vi "Save to CSV.vi"(8 "error in (no error)":errorcluster, 11 "Scan Data Process":T1) -> (0 "error out":errorcluster, 3 "Scan Data Process out":T1)   [LabVIEW 2015, in "Exposure Process.lvlib"]
uses:
  Exposure Process.lvlib
  Control_Scan Data Process.ctl
  <vilib>/addons/PointValueMap/controls/PointMap.ctl
  Control_EXP Information.ctl
  Control_File Save Setup.ctl
  Control_Enable and Path.ctl
  Control_ICM Export Setting.ctl
  FileHandler/controls/Record.ctl
  <vilib>/Utility/file.llb/Write Delimited Spreadsheet (string).vi
  FileHandler/FileHandler.lvlib
  <vilib>/addons/PointValueMap/PointValueMap.lvlib
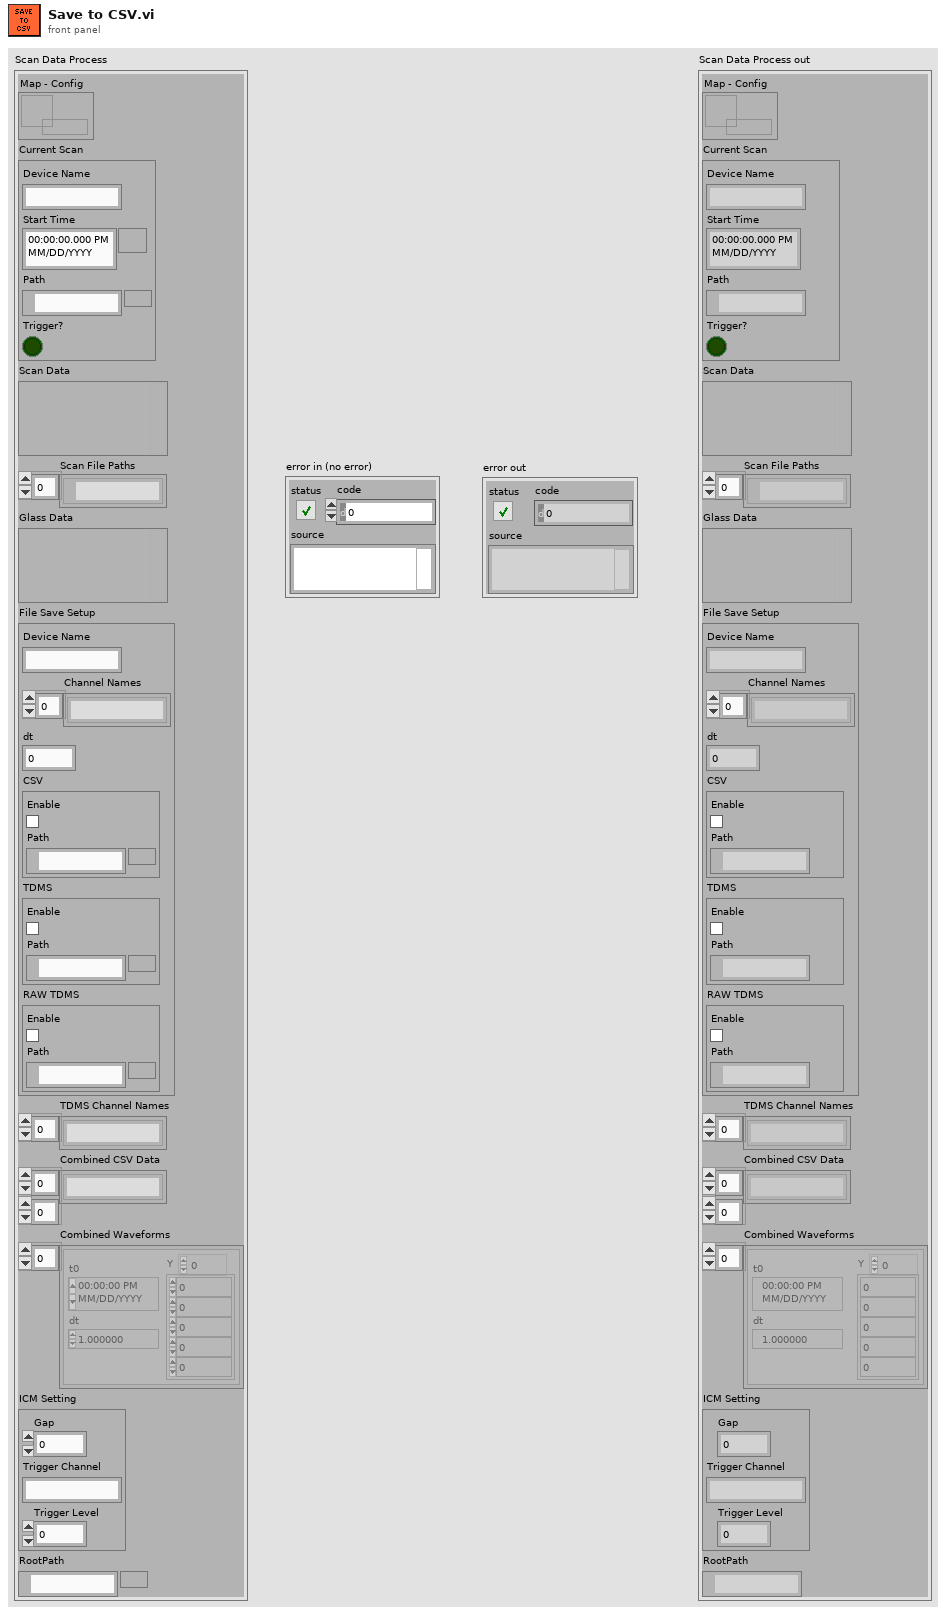
[diagram p1: front panel]
types:
  T1 = typedef "Exposure Process.lvlib/Control_Scan Data Process.ctl" = cluster{"Map - Config":T2, "Current Scan":T3, "Scan Data":variant, "Scan File Paths":path[], "Glass Data":variant, "File Save Setup":T4, "TDMS Channel Names":string[], "Combined CSV Data":string[][], "Combined Waveforms":waveform(dbl)[], "ICM Setting":T6, "RootPath":path}
  T2 = typedef "PointValueMap.lvlib/PointMap.ctl" = refnum<data-value>
  T3 = typedef "Exposure Process.lvlib/Control_EXP Information.ctl" = cluster{"Device Name":string, "Start Time":timestamp, "Path":path, "Trigger?":bool}
  T4 = typedef "Exposure Process.lvlib/Control_File Save Setup.ctl" = cluster{"Device Name":string, "Channel Names":string[], "dt":dbl, "CSV":T5, "TDMS":T5, "RAW TDMS":T5}
  T5 = typedef "Exposure Process.lvlib/Control_Enable and Path.ctl" = cluster{"Enable":bool, "Path":path}
  T6 = typedef "Exposure Process.lvlib/Control_ICM Export Setting.ctl" = cluster{"Gap":dbl, "Trigger Channel":string, "Trigger Level":dbl}
  T7 = typedef "FileHandler.lvlib/Record.ctl" = cluster{"Time":timestamp, "Path":path}
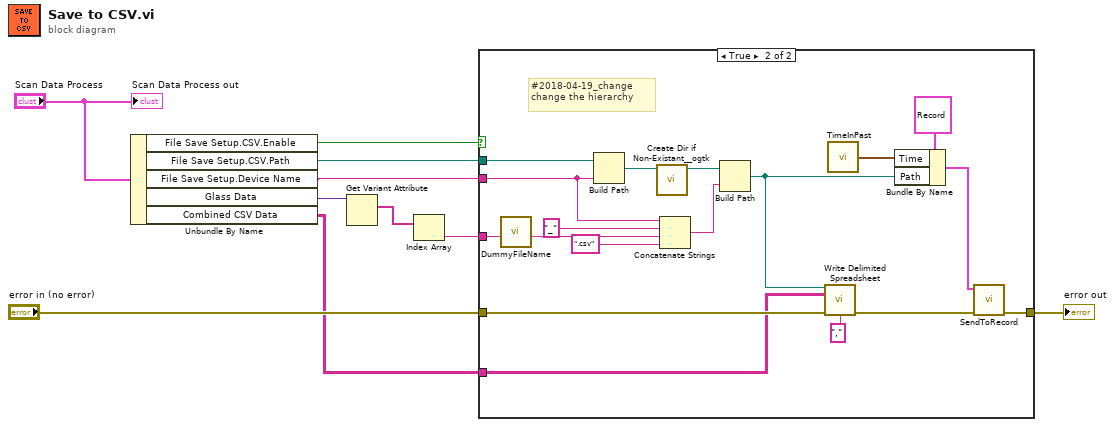
[diagram p0: block diagram]
diagram:
  n1 = Unbundle By Name("Scan Data Process") -> ("File Save Setup.CSV.Enable"=w9:bool, "File Save Setup.CSV.Path"=w8:path, "File Save Setup.Device Name"=w7:string, "Glass Data"=w4:variant, "Combined CSV Data"=w5:string[][])
  n2 = Get Variant Attribute(Variant=w4) -> (names=w3:string[])  [unwired: 3 in, 3 out]
  n3 = Index Array(array=w3) -> (element=w2:string)  [unwired: 1 in]
  n4 = case shown="True" w9 {
    tunnel: w2 -> [_ w14]
    tunnel: "error in (no error)" -> [w11 w25]
    tunnel: [w11 w18] -> w10
    tunnel: w5 -> [_ w23]
    tunnel: w8 -> [_ w22]
    tunnel: w7 -> [_ w20]
    frame False {
    }
    frame True {
      # "#2018-04-19_change\nchange the hierarchy"
      n5 = call "DummyFileName.vi"("Time String in"=w14) -> ("Time String out"=w13:string)  [unwired: 9 in, 1 out]
      n6 = Build Path(base path=w22, name or relative path=w20) -> (appended path=w21:path)
      n7 = call <userlib>:"Create Dir if Non-Existant__ogtk.vi"("Directory Path"=w21) -> ("dup Directory Path"=w26:path)  [unwired: 8 in, 2 out]
      n8 = Concatenate Strings(w20, "_" ("string"), w13, ".csv" ("string")) -> (w27:string)
      n9 = Build Path(base path=w26, name or relative path=w27) -> (appended path=w16:path)
      n10 = call-poly <vilib>:"Write Delimited Spreadsheet.vi"("file path (dialog if empty)"=w16, "2D data"=w23, "error in (no error)"=w25, "delimiter (\\t)"="," ("delimiter (\\t)")) -> ("error out"=w19:errorcluster)  [unwired: 10 in, 1 out]
      n11 = call "TimeInPast.vi"() -> ("Time Stamp"=w12:timestamp)
      n12 = Bundle By Name(cluster=T7 {"Time"=timestamp(0 s since 1904-01-01), "Path"=path ""} ("Record"), "Time"=w12, "Path"=w16) -> (w15:T7)
      n13 = call "SendToRecord.vi"("error in (no error)"=w19, "Record"=w15) -> ("error out"=w18:errorcluster)  [unwired: 9 in]
    }
  }
  "error out" <- w10
  "Scan Data Process out" <- "Scan Data Process"
